vi "Sprinkler.vi"() -> ()   [LabVIEW 2019]
uses:
  Controls/state machine enum.ctl
  Controls/Zone Indicators.ctl
  Controls/Controller Status.ctl
  Controls/Application Data.ctl
  Controls/Zone Setup Array.ctl
  Controls/Water Pressure Sensor.ctl
panel:
  out "error out":errorcluster
  in  "error in":errorcluster
  in  "Zone Setup Array":T1
  out "Controller Status":T2
  out "Zone Indicators":T3 {"Timing" format="%.4f"}
  in  "Water Pressure Sensor (%)":T4 scale=0.0..100.0
  in  "Rain Sensor":bool
  in  "Run Selector":bool
  in  "Setup":bool
  in  "Start":bool
  in  "stop":bool
  # "Controls"
  # "Simulation Controls"
  # "Rain"
  # "No Rain"
  # "Continuous"
  # "Single"
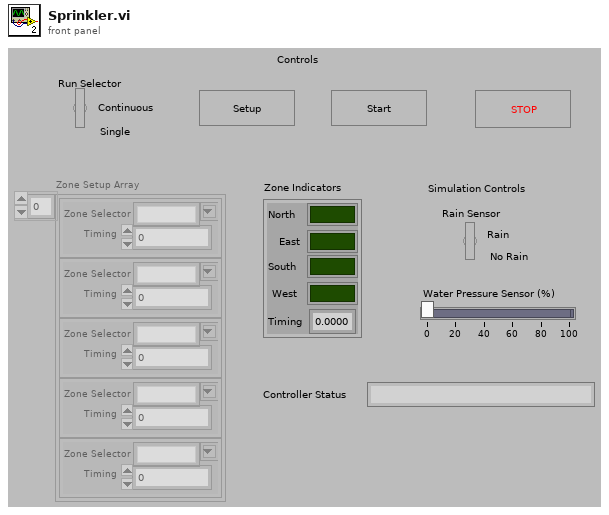
[diagram p1: front panel]
types:
  T1 = typedef "Zone Setup Array.ctl" = cluster{"Zone Selector":string, "Timing":dbl}[]
  T2 = typedef "Controller Status.ctl" = string
  T3 = typedef "Zone Indicators.ctl" = cluster{"North":bool, "East":bool, "South":bool, "West":bool, "Timing":sgl}
  T4 = typedef "Water Pressure Sensor.ctl" = u32
  T5 = typedef "Application Data.ctl" = cluster{"Zone Indicators":T3, "Controller Status":T2, "Zone Setup Array":T1, "Sprinkler running":bool, "Run Selector":bool, "Current zone index":i32, "Suspended":bool}
  T6 = typedef "state machine enum.ctl" = enum16{"Initialise", "Idle", "Load Program", "Run Sprinkler", "Exit"}
  T7 = enum16{"Get Time", "Reset Time", "Pause", "Resume"}
  T8 = enum8{"Enabled", "Disabled", "Disabled and Grayed Out"}
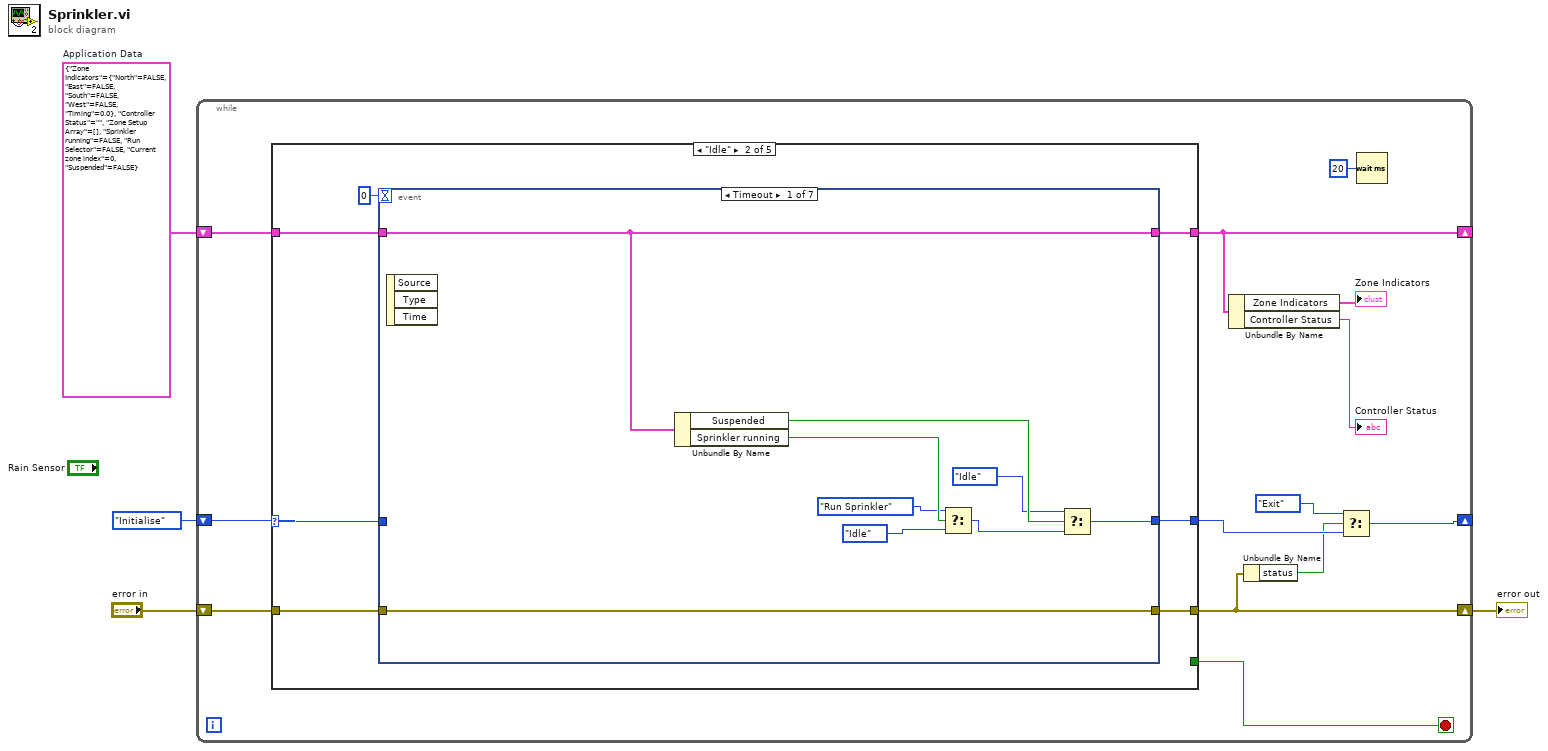
[diagram p0: block diagram]
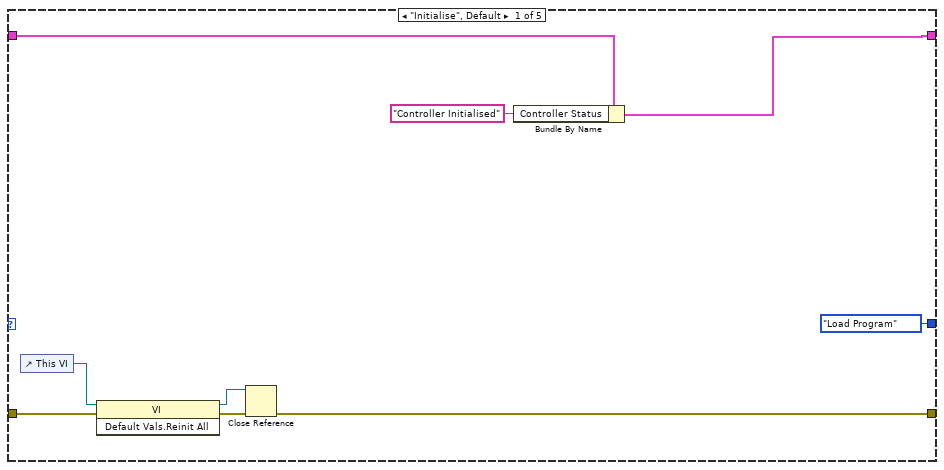
[diagram p2: hidden frame]
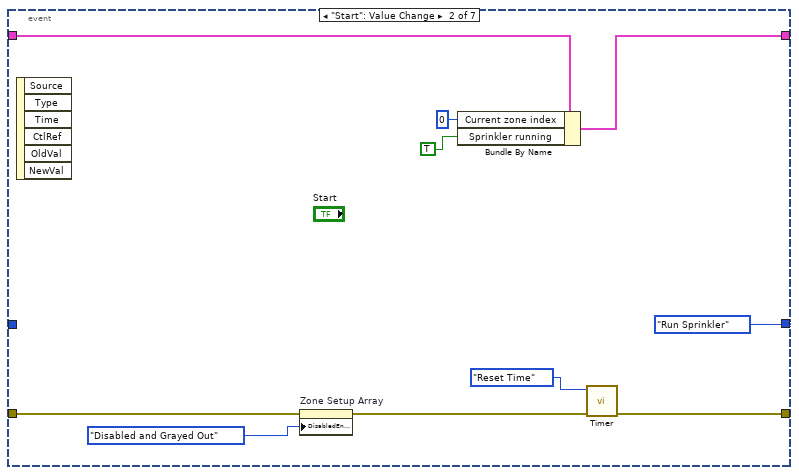
[diagram p3: hidden frame]
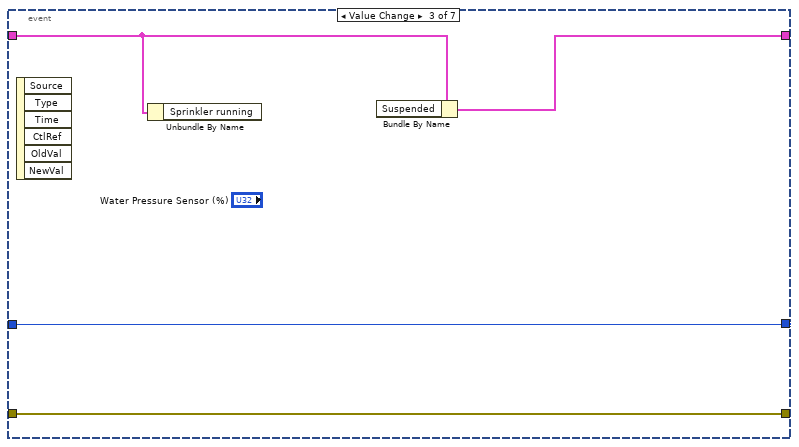
[diagram p4: hidden frame]
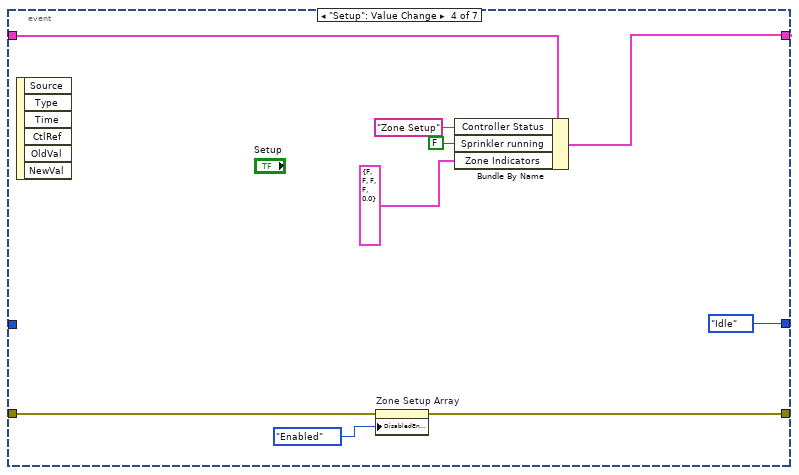
[diagram p5: hidden frame]
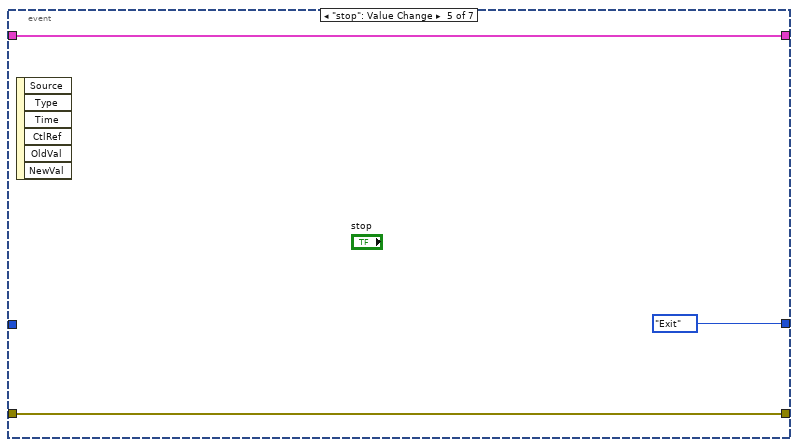
[diagram p6: hidden frame]
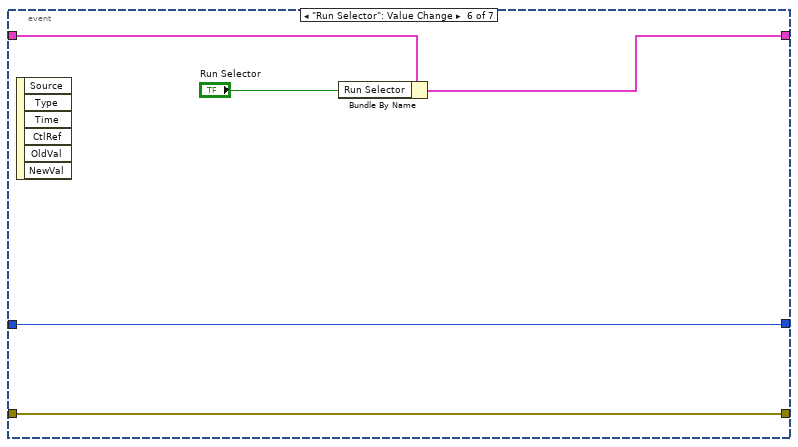
[diagram p7: hidden frame]
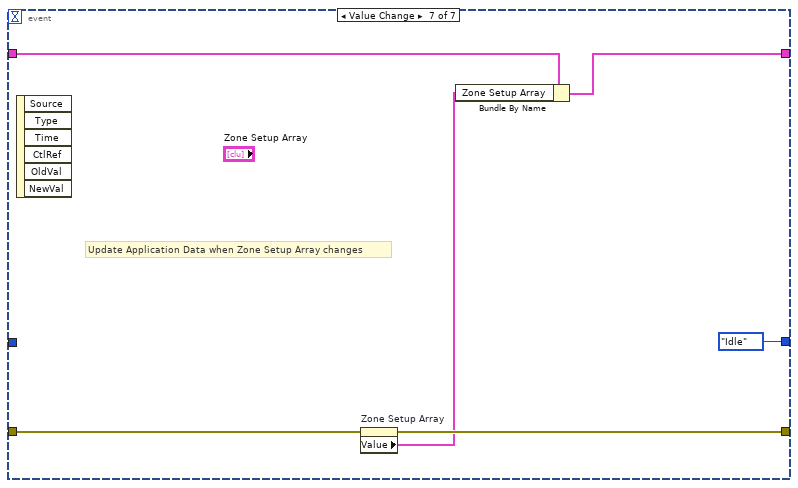
[diagram p8: hidden frame]
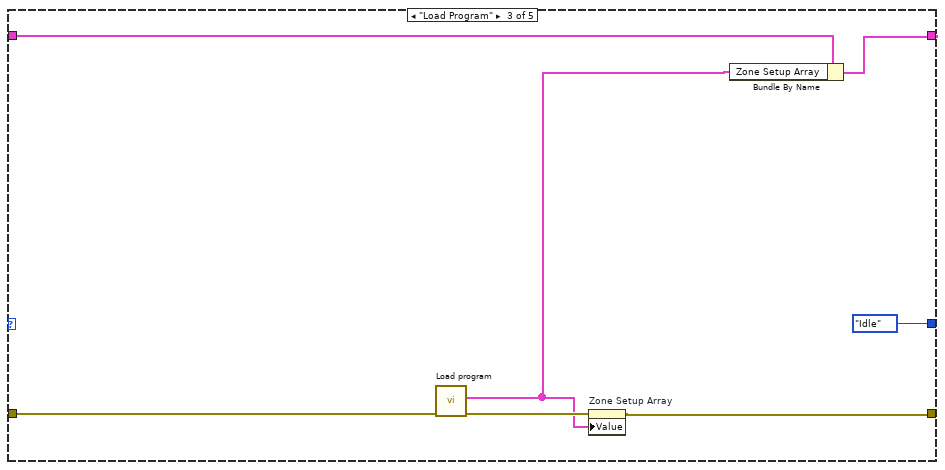
[diagram p9: hidden frame]
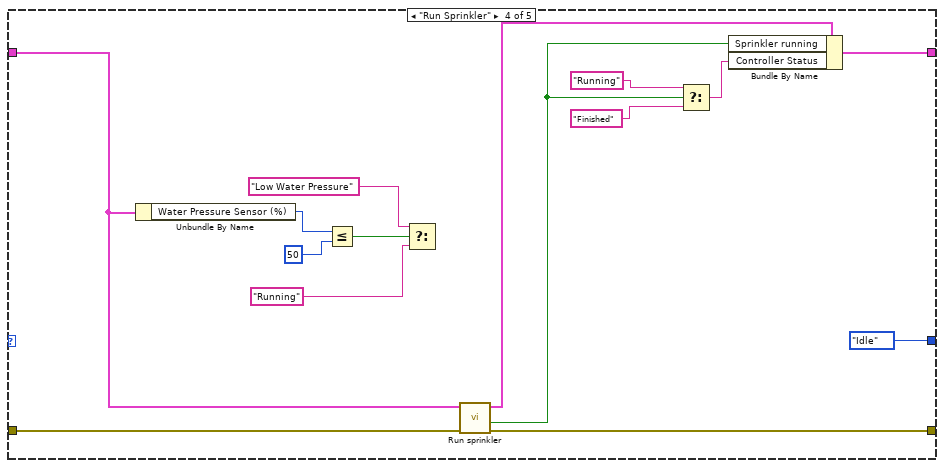
[diagram p10: hidden frame]
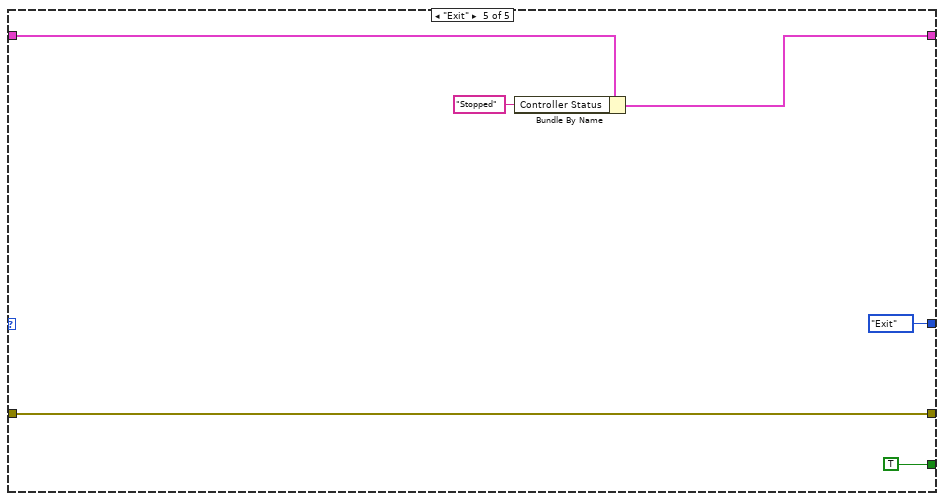
[diagram p11: hidden frame]
diagram:
  w1 = T5 {"Zone Indicators"={"North"=FALSE, "East"=FALSE, "South"=FALSE, "West"=FALSE, "Timing"=0.0}, "Controller Status"="", "Zone Setup Array"=[], "Sprinkler running"=FALSE, "Run Selector"=FALSE, "Current zone index"=0, "Suspended"=FALSE}  # Application Data
  n1 = while {
    shift-right: [w14] -> _
    shift-left: state_machine_enum."Initialise" -> [w17]
    shift-right: [w12] -> w2
    shift-left: "error in" -> [w16]
    shift-right: [w8] -> _
    shift-left: w1 -> [w9]
    stop <- w10 stop-if-true
    n2 = case shown="\"Idle\"" w17 {
      selector: w17 -> [_ w33 _ _ _]
      tunnel: [state_machine_enum."Load Program" w32 state_machine_enum."Idle" state_machine_enum."Idle" state_machine_enum."Exit"] -> w15
      tunnel: w16 -> [w25 w31 w86 w93 w107]
      tunnel: [w21 w30 w80 w94 w107] -> w12
      tunnel: [_ _ _ _ TRUE] -> w10
      tunnel: w9 -> [w20 w29 w85 w95 w104]
      tunnel: [w19 w28 w84 w91 w103] -> w8
      frame "Initialise", Default {
        n3 = control-ref of="This VI"() -> (w26:refnum<vi>)
        n4 = invoke class="VI" method="Default Vals.Reinit All"(reference=w26, error in=w25) -> (reference out=w22:refnum<vi>, error out=w23:errorcluster)  [unwired: 1 in, 1 out]
        n5 = Close Reference(reference=w22, error in (no error)=w23) -> (error out=w21:errorcluster)
        n6 = Bundle By Name(cluster=w20, "Controller Status"=T2 "Controller Initialised") -> (w19:T5)
      }
      frame "Idle" {
        n7 = event shown="[0] Timeout" {
          selector: _ -> [_ _ _ _ _ _ _]
          dyn-events: _ -> [_ _ _ _ _ _ _]
          timeout: 0 -> [_ _ _ _ _ _ _]
          tunnel: w33 -> [_ _ w55 _ _ w73 _]
          tunnel: [w36 state_machine_enum."Run Sprinkler" w55 state_machine_enum."Idle" state_machine_enum."Exit" w73 state_machine_enum."Idle"] -> w32
          tunnel: w31 -> [w42 w50 w54 w65 w68 w72 w79]
          tunnel: [w42 w43 w54 w64 w68 w72 w78] -> w30
          tunnel: w29 -> [w41 w49 w53 w61 w66 w71 w77]
          tunnel: [w41 w48 w56 w59 w66 w70 w76] -> w28
          event Timeout {
            n8 = event-data() -> ()  [unwired: 1 in, 3 out]
            n9 = Unbundle By Name(w41) -> ("Suspended"=w35:bool, "Sprinkler running"=w40:bool)
            n10 = Select(t=state_machine_enum."Run Sprinkler", s=w40, f=state_machine_enum."Idle") -> (s? t:f=w37:T6)
            n11 = Select(t=state_machine_enum."Idle", s=w35, f=w37) -> (s? t:f=w36:T6)
          }
          event "Start": Value Change {
            n12 = event-data() -> ()  [unwired: 1 in, 6 out]
            n13 = property on="Zone Setup Array" class="Arr (strict)"(error in=w50, "DisabledEnum"=T8."Disabled and Grayed Out" ("Disabled")) -> (error out=w44:errorcluster)  [unwired: 1 in, 1 out]
            n14 = Bundle By Name(cluster=w49, "Current zone index"=0, "Sprinkler running"=TRUE ("Sprinkler running?")) -> (w48:T5)
            n15 = call "Timer.vi"("error in (no error)"=w44, "Enum"=T7."Reset Time") -> ("error out"=w43:errorcluster)  [unwired: 8 in, 1 out]
          }
          event Value Change {
            n16 = event-data() -> ()  [unwired: 1 in, 6 out]
            n17 = Unbundle By Name(w53) -> ()  [unwired: 1 out]
            n18 = Bundle By Name(cluster=w53) -> (w56:T5)  [unwired: 1 in]
          }
          event "Setup": Value Change {
            n19 = event-data() -> ()  [unwired: 1 in, 6 out]
            n20 = property on="Zone Setup Array" class="Arr (strict)"(error in=w65, "DisabledEnum"=T8."Enabled" ("Disabled")) -> (error out=w64:errorcluster)  [unwired: 1 in, 1 out]
            n21 = Bundle By Name(cluster=w61, "Controller Status"=T2 "Zone Setup", "Sprinkler running"=FALSE ("Sprinkler running?"), "Zone Indicators"=T3 {"North"=FALSE, "East"=FALSE, "South"=FALSE, "West"=FALSE, "Timing"=0.0}) -> (w59:T5)
          }
          event "stop": Value Change {
            n22 = event-data() -> ()  [unwired: 1 in, 6 out]
          }
          event "Run Selector": Value Change {
            n23 = event-data() -> ()  [unwired: 1 in, 6 out]
            n24 = Bundle By Name(cluster=w71, "Run Selector"="Run Selector") -> (w70:T5)
          }
          event Value Change {
            # "Update Application Data when Zone Setup Array changes"
            n25 = event-data() -> ()  [unwired: 1 in, 6 out]
            n26 = property on="Zone Setup Array" class="Arr (strict)"(error in=w79) -> (error out=w78:errorcluster, "Value"=w75:T1)  [unwired: 1 in, 1 out]
            n27 = Bundle By Name(cluster=w77, "Zone Setup Array"=w75) -> (w76:T5)
          }
        }
      }
      frame "Load Program" {
        n28 = call "Load program.vi"("error in"=w86) -> ("error out"=w82:errorcluster, "Zone Setup Array Data"=w81:T1)  [unwired: 9 in]
        n29 = property on="Zone Setup Array" class="Arr (strict)"(error in=w82, "Value"=w81) -> (error out=w80:errorcluster)  [unwired: 1 in, 1 out]
        n30 = Bundle By Name(cluster=w85, "Zone Setup Array"=w81) -> (w84:T5)
      }
      frame "Run Sprinkler" {
        n31 = Unbundle By Name(w95) -> ("Water Pressure Sensor (%)"=w99:T4)
        n32 = Less Or Equal?(x=w99, y=u32 50) -> (x <= y?=w97:bool)
        n33 = Select(t="Low Water Pressure" ("Controller Status"), s=w97, f="Running" ("Controller Status")) -> ()  [unwired: 1 out]
        n34 = call "Run sprinkler.vi"("error in (no error)"=w93, "Application Data"=w95) -> ("error out"=w94:errorcluster, "Sprinkler running?"=w90:bool, "Application Data 2"=w92:T5)  [unwired: 7 in]
        n35 = Select(t="Running", s=w90, f="Finished") -> (s? t:f=w89:string)
        n36 = Bundle By Name(cluster=w92, "Sprinkler running"=w90, "Controller Status"=w89) -> (w91:T5)
      }
      frame "Exit" {
        n37 = Bundle By Name(cluster=w104, "Controller Status"=T2 "Stopped") -> (w103:T5)
      }
    }
    n38 = Unbundle By Name(w8) -> ("Zone Indicators"=→"Zone Indicators":T3, "Controller Status"=→"Controller Status":T2)
    n39 = Unbundle By Name(w12) -> ("status"=w11:bool)
    n40 = Select(t=state_machine_enum."Exit", s=w11, f=w15) -> (s? t:f=w14:T6)
    n41 = Wait (ms)(milliseconds to wait=u32 20) -> ()  [unwired: 1 out]
  }
  "error out" <- w2
